vi "CRC_Check.vi"(8 "Mode simulation":bool, 9 "CRC attendu simulation":i32=142, 10 "CRC recu":i32, 11 "Trame":string) -> (3 "CRC valide":bool)   [LabVIEW 2022 SP3]
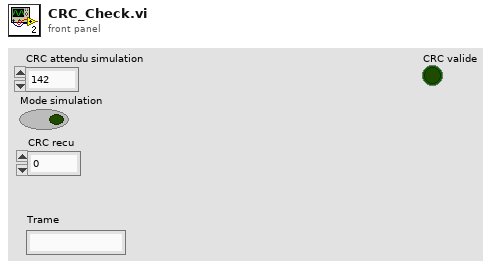
[diagram p1: front panel]
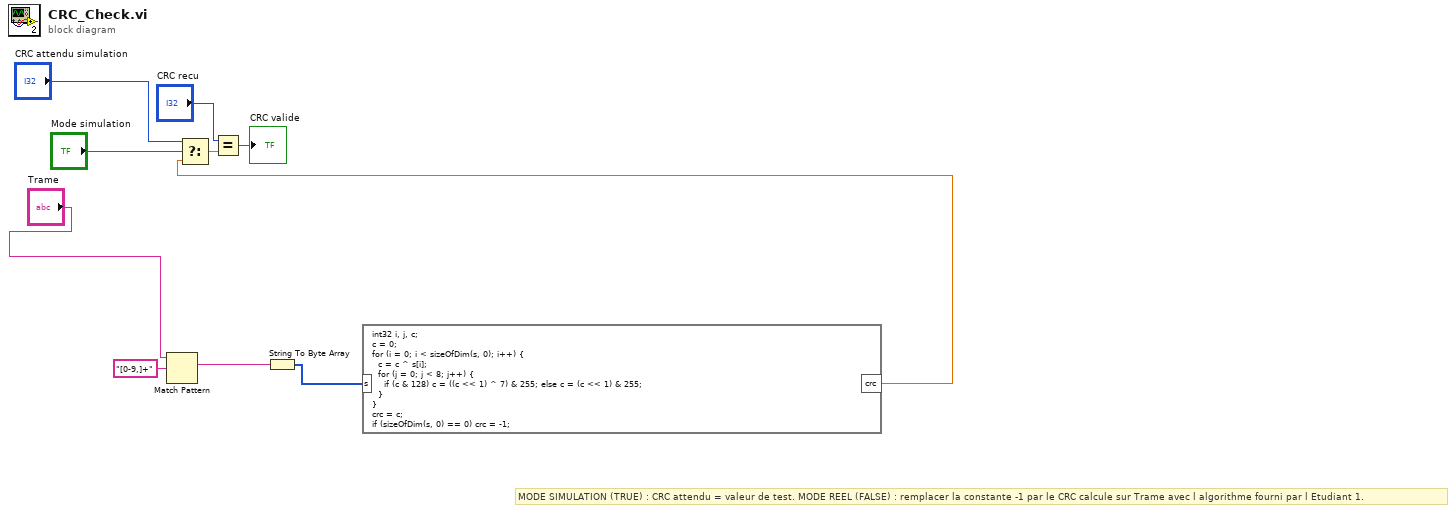
[diagram p0: block diagram]
diagram:
  # "MODE SIMULATION (TRUE) : CRC attendu = valeur de test. MODE REEL (FALSE) : remplacer la constante -1 par le CRC calcule sur Trame avec l algorithme fourni par l Etudiant 1."
  n1 = Match Pattern(string="Trame", regular expression="[0-9,]+") -> (match substring=w1:string)  [unwired: 1 in, 3 out]
  n2 = String To Byte Array(string=w1) -> (unsigned byte array=w5:u8[])
  n3 = formula code="int32 i, j, c;\nc = 0;\nfor (i = 0; i < sizeOfDim(s, 0); i++) {\n  c = c ^ s[i];\n  for (j = 0; j < 8; j++) {\n    if (c & 128) c = ((c << 1) ^ 7) & 255; else c = (c << 1) & 255;\n  }\n}\ncrc = c;\nif (sizeOfDim(s, 0) == 0) crc = -1;"("s"=w5) -> ("crc"=w4:dbl)
  n4 = Select(t="CRC attendu simulation", s="Mode simulation", f=w4) -> (s? t:f=w10:dbl)
  n5 = Equal?(x="CRC recu", y=w10) -> (x = y?=→"CRC valide":bool)
